vi "Limelight_To_Turret.vi"(8 "lower limit":dbl=-512.0 format="%#_13g", 9 "Limelight X":dbl(knob) scale=-5.0..5.0, 10 "Current":dbl(knob) scale=-7100.0..6800.0, 11 "upper limit":dbl=512.0 format="%#_13g") -> (3 "OutputForTurret":dbl(knob) scale=-7100.0..6800.0)   [LabVIEW 2019]
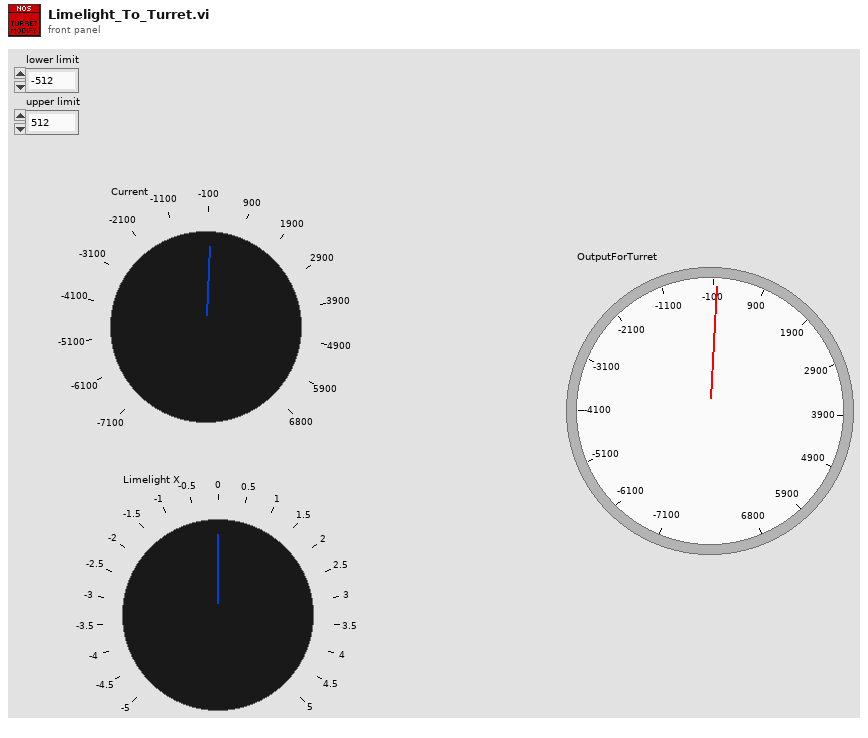
[diagram p1: front panel]
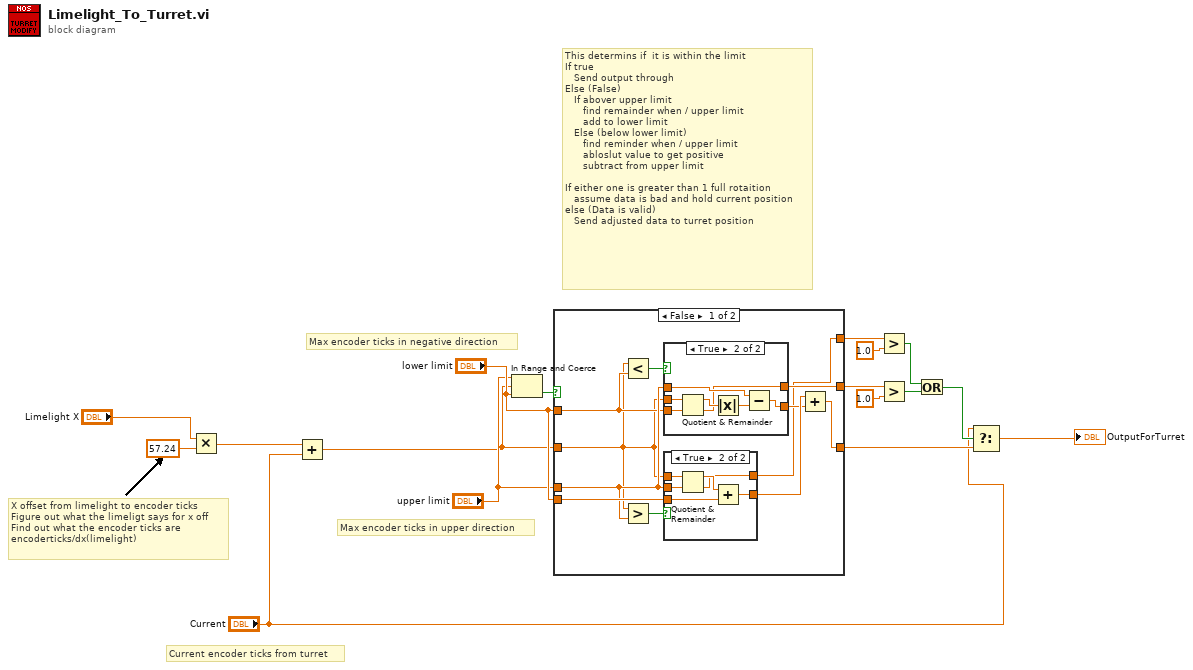
[diagram p0: block diagram]
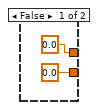
[diagram p2: hidden frame]
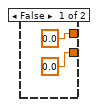
[diagram p3: hidden frame]
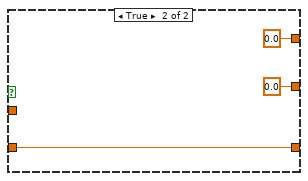
[diagram p4: hidden frame]
diagram:
  # "Current encoder ticks from turret"
  # "Max encoder ticks in upper direction"
  # "Max encoder ticks in negative direction"
  # "This determins if  it is within the limit\nIf true\n   Send output through\nElse (False)\n   If abover upper limit\n      find remainder when / upper limit\n      add to lower limit\n   Else (below lower limit)\n      find reminder when / upper limit\n      abloslut value to get positive\n      subtract from upper limit\n\nIf either one is greater than 1 full rotaition\n   assume data is bad and hold current position\nelse (Data is valid)\n   Send adjusted data to turret position"
  # "X offset from limelight to encoder ticks\nFigure out what the limeligt says for x off\nFind out what the encoder ticks are\nencoderticks/dx(limelight)"
  n1 = Multiply(x="Limelight X", y=57.24) -> (x*y=w5:dbl)
  n2 = Add(x=w5, y="Current") -> (x+y=w3:dbl)
  n3 = In Range and Coerce(upper limit="upper limit", x=w3, lower limit="lower limit") -> (In Range?=w17:bool)  [unwired: 1 out]
  n4 = case shown="False" w17 {
    tunnel: [w26 w48] -> w8
    tunnel: w3 -> [w20 w48]
    tunnel: "upper limit" -> [w22 _]
    tunnel: "lower limit" -> [w21 _]
    tunnel: "lower limit" -> [w23 _]
    tunnel: [w19 0.0] -> w15
    tunnel: [w18 0.0] -> w12
    frame False {
      n5 = Less?(x=w20, y=w21) -> (x < y?=w27:bool)
      n6 = Greater?(x=w20, y=w22) -> (0:w28:bool)
      n7 = case shown="True" w27 {
        tunnel: [0.0 ("lower limit") w32] -> w24
        tunnel: w20 -> [_ w36]
        tunnel: w22 -> [_ w33]
        tunnel: w21 -> [_ w37]
        tunnel: [0.0 w31] -> w19
        frame False {
        }
        frame True {
          n8 = Quotient & Remainder(x=w36, y=w37) -> (x-y*floor(x/y)=w35:dbl, floor(x/y)=w31:dbl)
          n9 = Absolute Value(x=w35) -> (abs(x)=w34:dbl)
          n10 = Subtract(x=w33, y=w34) -> (x-y=w32:dbl)
        }
      }
      n11 = case shown="True" w28 {
        tunnel: [0.0 ("lower limit") w41] -> w25
        tunnel: w22 -> [_ w45]
        tunnel: w20 -> [_ w44]
        tunnel: w23 -> [_ w43]
        tunnel: [0.0 w40] -> w18
        frame False {
        }
        frame True {
          n12 = Quotient & Remainder(x=w44, y=w45) -> (x-y*floor(x/y)=w42:dbl, floor(x/y)=w40:dbl)
          n13 = Add(x=w42, y=w43) -> (x+y=w41:dbl)
        }
      }
      n14 = Add(x=w25, y=w24) -> (x+y=w26:dbl)
    }
    frame True {
    }
  }
  n15 = Greater?(x=w12, y=1.0) -> (0:w10:bool)
  n16 = Greater?(x=w15, y=1.0) -> (0:w11:bool)
  n17 = Or(x=w10, y=w11) -> (x .or. y?=w9:bool)
  n18 = Select(t="Current", s=w9, f=w8) -> (s? t:f=→"OutputForTurret":dbl)
